vi "Subvi buffer pixel clock.vi"   [LabVIEW 2017]
uses:
  <vilib>/rvi/Emulation/niFpgaSctlEmulationGetInTimedLoop.vi
  GV FIFO timeout.vi
  <vilib>/rvi/interface/RandomDataEmulation/niFpgaRandomDataHandleErrors.vi
  Detector/GV N pixel clock per line.vi
  <vilib>/rvi/Emulation/niFpgaProcessEmulError.vi
  <vilib>/rvi/Memory/Memory_Emulation/nirvimemoryFastEmulation.vi
  <vilib>/rvi/Memory/Memory_Emulation/nirvimemoryEmulation.vi
  <vilib>/rvi/Emulation/niFpgaEmulationIsFPGAContextNoSignature.vi
  <vilib>/rvi/DataTransferAndStorage/Container/Common/niFpgaContainerGetUniqueNameForEmu.vi
  <vilib>/rvi/errors/nirviReportUnexpectedCaseInternalError (U32).vi
  <vilib>/rvi/DataTransferAndStorage/Container/XNode/niFpgaContainer.xnode
  <vilib>/rvi/interface/RandomDataEmulation/nirviRandomDataFpgaReadWriteTemplate.vi
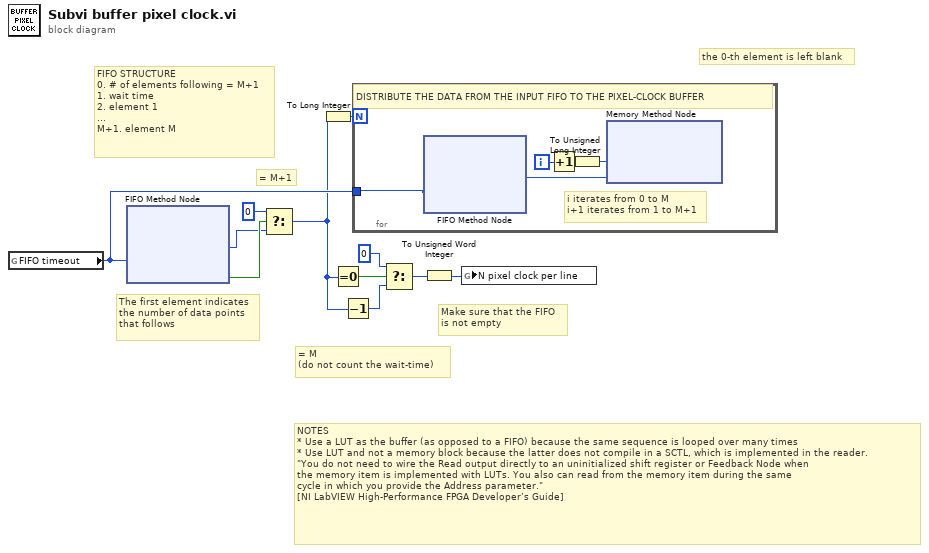
[diagram p0: block diagram]
diagram:
  # "Make sure that the FIFO\nis not empty"
  # "= M\n(do not count the wait-time)"
  # "the 0-th element is left blank"
  # "NOTES\n* Use a LUT as the buffer (as opposed to a FIFO) because the same sequence is looped over many times\n* Use LUT and not a memory block because the latter does not compile in a SCTL, which is implemented in the reader.\n\"You do not need to wire the Read output directly to an uninitialized shift register or Feedback Node when\nthe memory item is implemented with LUTs. You also can read from the memory item during the same\ncycle in which you provide the Address parameter.\"\n[NI LabVIEW High-Performance FPGA Developer’s Guide]"
  # "FIFO STRUCTURE\n0. # of elements following = M+1\n1. wait time\n2. element 1\n...\nM+1. element M"
  # "= M+1"
  # "The first element indicates\nthe number of data points\nthat follows"
  n1 = global read "GV FIFO timeout.vi" "FIFO timeout"() -> (w10:i32)
  n2 = xnode ("FIFO Method Node")("Timeout"=w10) -> ("Element"=w8:u32, "Timed Out?"=w9:bool)  [unwired: 1 in, 1 out]
  n3 = Select(t=u32 0, s=w9, f=w8) -> (s? t:f=w3:u32)
  n4 = To Long Integer(number=w3) -> (32bit integer=w7:i32)
  n5 = Equal To 0?(x=w3) -> (x = 0?=w5:bool)
  n6 = Decrement(x=w3) -> (x-1=w2:u32)
  n7 = for {
    N: w7 -> [_]
    tunnel: w10 -> [w16]
    i -> [w15]
    # "i iterates from 0 to M\ni+1 iterates from 1 to M+1"
    # "DISTRIBUTE THE DATA FROM THE INPUT FIFO TO THE PIXEL-CLOCK BUFFER"
    n8 = xnode ("FIFO Method Node")("Timeout"=w16) -> ("Element"=w12:u32)  [unwired: 1 in, 2 out]
    n9 = Increment(x=w15) -> (x+1=w14:i32)
    n10 = To Unsigned Long Integer(number=w14) -> (unsigned 32bit integer=w13:u32)
    n11 = xnode ("Memory Method Node")("Address"=w13, "Data"=w12) -> ()  [unwired: 1 in, 1 out]
  }
  n12 = Select(t=u32 0, s=w5, f=w2) -> (s? t:f=w1:u32)
  n13 = To Unsigned Word Integer(number=w1) -> (unsigned 16bit integer=w6:u16)
  n14 = global write "GV N pixel clock per line.vi" "N pixel clock per line"(w6) -> ()
